vi "WS1050_AD7747_Init.vi"(8 "error in":errorcluster) -> (0 "error out":errorcluster)   [LabVIEW 2012]
panel:
  # "Initialize AD7747 for Capacitance Measurement Mode"
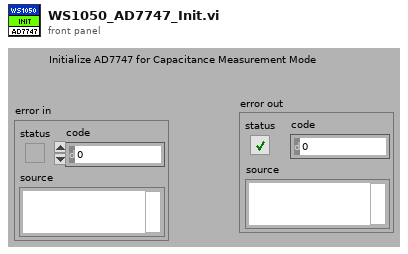
[diagram p1: front panel]
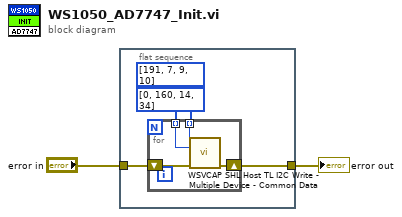
[diagram p0: block diagram]
diagram:
  n1 = flat-sequence {
    tunnel: "error in" -> [w4]
    tunnel: [w3] -> w2
    frame #0 {
      n2 = for {
        tunnel: u8[] [191, 7, 9, 10] -> [w10] mode=indexing
        tunnel: u8[] [0, 160, 14, 34] -> [w9] mode=indexing
        shift-right: [w8] -> w3
        shift-left: w4 -> [w7]
        n3 = call "WSVCAP SHL Host TL I2C Write - Multiple Device - Common Data.vi"("Sub Address"=w10, "Data Out [U8]"=w9, "error in"=w7) -> ("error out"=w8:errorcluster)  [unwired: 12 in]
      }
    }
  }
  "error out" <- w2
